vi "Unit Test.vi"() -> ()   [LabVIEW 2019, in "NE-500.lvlib"]
uses:
  NE-500.lvlib
  User Event/Controls/UE Abort Action.ctl
panel:
  out "Status":string
  in  "Read Stop":bool
  in  "Read":bool
  in  "VISA name":refnum<visa-resource-name>="visa://169.254.25.118/ASRL2::INSTR"
  in  "Initialize":bool
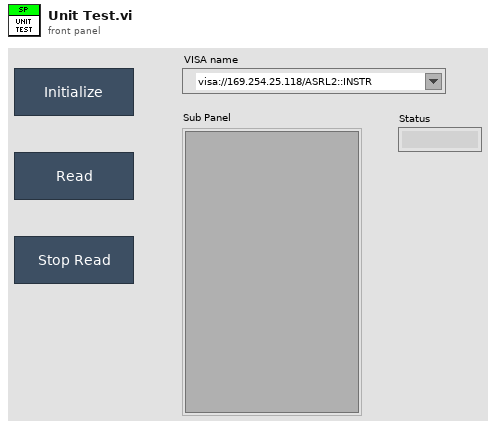
[diagram p1: front panel]
types:
  T1 = typedef "UE Abort Action.ctl" = enum16{"Create", "Get", "Destroy"}
  T2 = typedef "NE-500.lvlib/SEQ Data.ctl" = cluster{"Status":string, "Initialize Done?":bool, "VI Refnum":refnum<vi>}
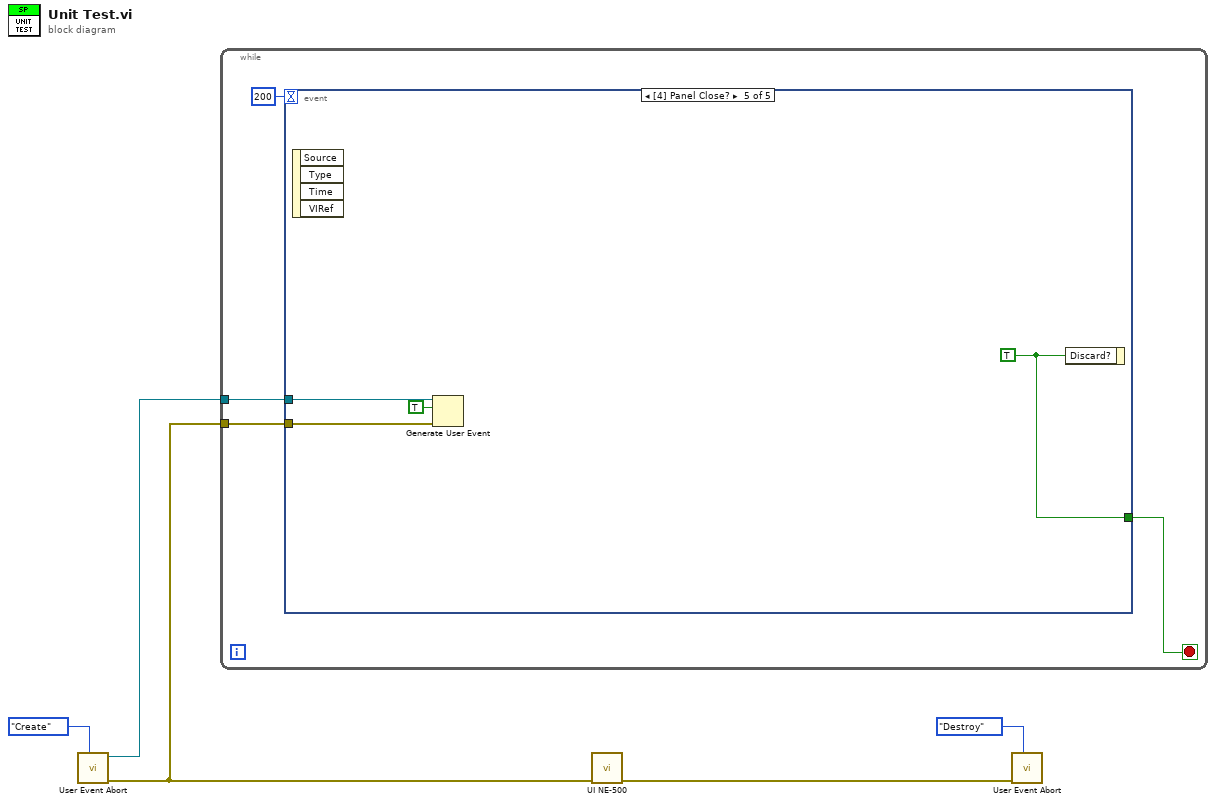
[diagram p0: block diagram]
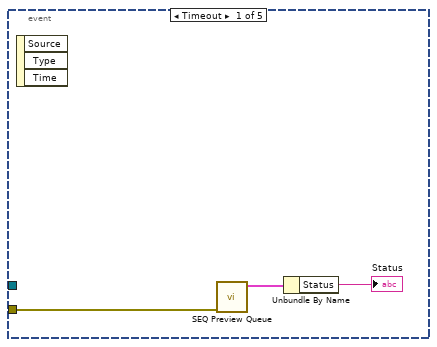
[diagram p2: hidden frame]
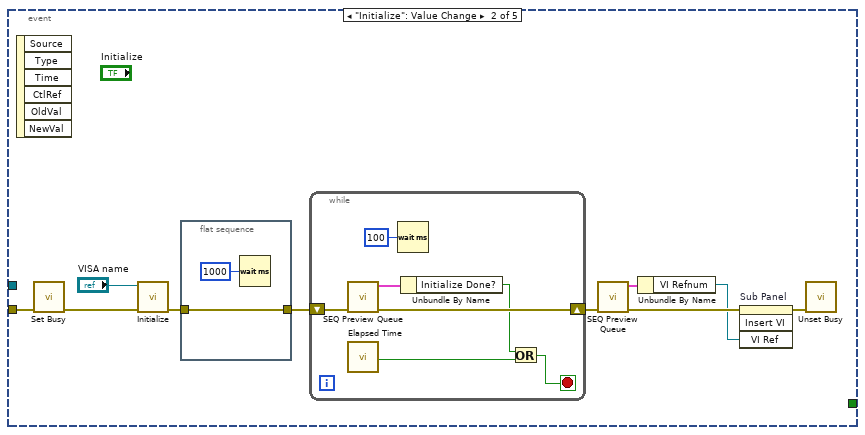
[diagram p3: hidden frame]
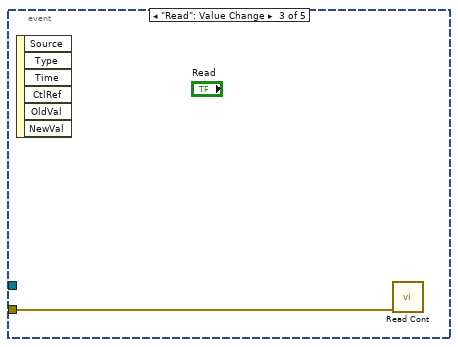
[diagram p4: hidden frame]
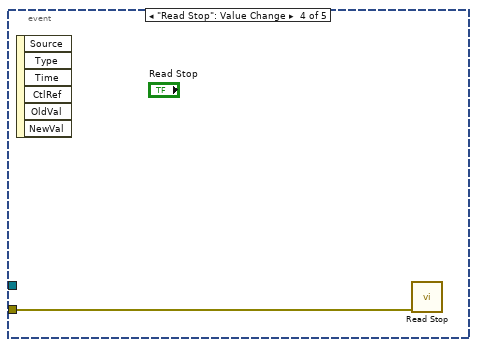
[diagram p5: hidden frame]
diagram:
  n1 = call "User Event Abort.vi"("Action"=UE_Abort_Action."Create") -> ("Error Out"=w1:errorcluster, "User Event Out"=w2:refnum<user-event>)  [unwired: 9 in]
  n2 = while {
    tunnel: w2 -> [w9]
    tunnel: w1 -> [w8]
    stop <- w7 stop-if-true
    n3 = event shown="[4] Panel Close?" {
      selector: _ -> [_ _ _ _ _]
      dyn-events: _ -> [_ _ _ _ _]
      timeout: 200 -> [_ _ _ _ _]
      tunnel: w9 -> [_ _ _ _ w36]
      tunnel: w8 -> [w12 w22 w32 w33 w35]
      tunnel: [_ _ _ _ w37] -> w7
      event Timeout {
        n4 = event-data() -> ()  [unwired: 1 in, 3 out]
        n5 = call "SEQ Preview Queue.vi"("error in"=w12) -> ("SEQ Data"=w11:T2)  [unwired: 9 in, 1 out]
        n6 = Unbundle By Name(w11) -> ("Status"=→"Status":string)
      }
      event "Initialize": Value Change {
        n7 = event-data() -> ()  [unwired: 1 in, 6 out]
        n8 = call <vilib>:"Set Busy.vi"("error in (no error)"=w22) -> ("error out"=w21:errorcluster)  [unwired: 9 in, 1 out]
        n9 = call "Initialize.vi"("Error In"=w21, "VISA name"="VISA name") -> ("Error Out"=w19:errorcluster)  [unwired: 9 in]
        n10 = flat-sequence {
          tunnel: w19 -> [w31]
          tunnel: [w31] -> w18
          frame #0 {
            n11 = Wait (ms)(milliseconds to wait=u32 1000) -> ()  [unwired: 1 out]
          }
        }
        n12 = while {
          shift-right: [w27] -> w17
          shift-left: w18 -> [w29]
          stop <- w23 stop-if-true
          n13 = call "SEQ Preview Queue.vi"("error in"=w29) -> ("error out"=w27:errorcluster, "SEQ Data"=w28:T2)  [unwired: 9 in]
          n14 = call "Elapsed Time"() -> ("Time has Elapsed"=w24:bool)  [unwired: 12 in, 7 out]
          n15 = Wait (ms)(milliseconds to wait=u32 100) -> ()  [unwired: 1 out]
          n16 = Unbundle By Name(w28) -> ("Initialize Done?"=w25:bool)
          n17 = Or(x=w25, y=w24) -> (x .or. y?=w23:bool)
        }
        n18 = call "SEQ Preview Queue.vi"("error in"=w17) -> ("error out"=w15:errorcluster, "SEQ Data"=w16:T2)  [unwired: 9 in]
        n19 = Unbundle By Name(w16) -> ("VI Refnum"=w13:refnum<vi>)
        n20 = invoke on="Sub Panel" class="SubPnl" method="Insert VI"(error in=w15, "VI Ref"=w13) -> (error out=w14:errorcluster)  [unwired: 2 in, 3 out]
        n21 = call <vilib>:"Unset Busy.vi"("error in (no error)"=w14) -> ()  [unwired: 10 in, 1 out]
      }
      event "Read": Value Change {
        n22 = event-data() -> ()  [unwired: 1 in, 6 out]
        n23 = call "Read Cont.vi"("Error In"=w32) -> ()  [unwired: 10 in, 1 out]
      }
      event "Read Stop": Value Change {
        n24 = event-data() -> ()  [unwired: 1 in, 6 out]
        n25 = call "Read Stop.vi"("Error In"=w33) -> ()  [unwired: 10 in, 1 out]
      }
      event Panel Close? {
        w37 = TRUE
        n26 = event-data() -> ()  [unwired: 1 in, 4 out]
        n27 = Generate User Event(user event=w36, event data cluster=TRUE ("event data"), error in=w35) -> ()  [unwired: 1 in, 2 out]
        n28 = event-data("Discard?"=w37) -> ()  [unwired: 1 in, 1 out]
      }
    }
  }
  n29 = call "UI NE-500.vi"("error in"=w1) -> ("error out"=w3:errorcluster)  [unwired: 10 in]
  n30 = call "User Event Abort.vi"("Action"=UE_Abort_Action."Destroy", "Error In"=w3) -> ()  [unwired: 8 in, 2 out]
